vi "IMAQ ROI Type to MSC ROI Type.vi"(0 "IMAQ ROI Type":u32(ring)=4 items=["No Selection", "Point", "Line", "Rectangle", "Oval", "Polygon", "Freehand Region", "Annulus", "Unused2", "Unused3", "Broken Line", "Freehand Line", "Rotated Rectangle"], 11 "error in (no error)":errorcluster) -> (4 "MSC ROI Type":T1 items=["Point", "Line", "Rectangle", "Oval", "Freehand / Polygon"], 15 "error out":errorcluster)   [LabVIEW 2014]
doc: "Conversion from MSC Picture type to IMAQ type"
uses:
  MSC Image_class/controls/ROI Type.ctl
  MSC Image_class/MSC Image.lvclass
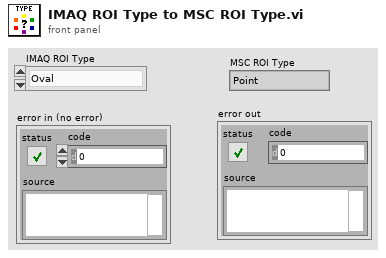
[diagram p1: front panel]
types:
  T1 = typedef "MSC Image.lvclass/ROI Type.ctl" = u16
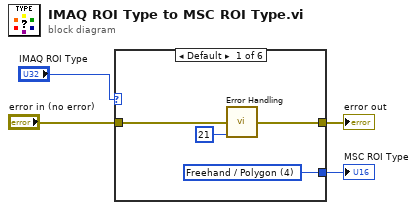
[diagram p0: block diagram]
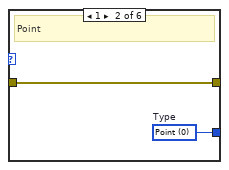
[diagram p2: hidden frame]
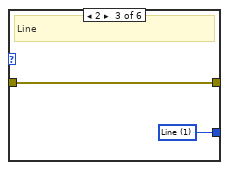
[diagram p3: hidden frame]
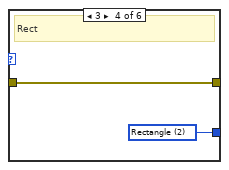
[diagram p4: hidden frame]
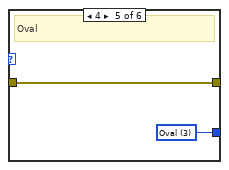
[diagram p5: hidden frame]
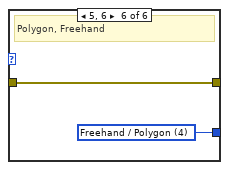
[diagram p6: hidden frame]
diagram:
  n1 = case shown="Default" "IMAQ ROI Type" {
    tunnel: "error in (no error)" -> [w5 w10 w12 w14 w15 w18]
    tunnel: [w6 w10 w12 w14 w15 w18] -> w2
    tunnel: [w8 w9 w11 w13 w16 w17] -> w3
    frame Default {
      w8 = T1 4 items=["Point", "Line", "Rectangle", "Oval", "Freehand / Polygon"] ("Type")
      n2 = call "Error Handling.vi"("error in (no error)"=w5, "return type"=21 ("code")) -> ("error out"=w6:errorcluster)  [unwired: 12 in, 1 out]
    }
    frame 1 {
      w9 = T1 0 items=["Point", "Line", "Rectangle", "Oval", "Freehand / Polygon"]  # Type
      # "Point"
    }
    frame 2 {
      w11 = T1 1 items=["Point", "Line", "Rectangle", "Oval", "Freehand / Polygon"] ("Type")
      # "Line"
    }
    frame 3 {
      w13 = T1 2 items=["Point", "Line", "Rectangle", "Oval", "Freehand / Polygon"] ("Type")
      # "Rect"
    }
    frame 4 {
      w16 = T1 3 items=["Point", "Line", "Rectangle", "Oval", "Freehand / Polygon"] ("Type")
      # "Oval"
    }
    frame 5, 6 {
      w17 = T1 4 items=["Point", "Line", "Rectangle", "Oval", "Freehand / Polygon"] ("Type")
      # "Polygon, Freehand"
    }
  }
  "error out" <- w2
  "MSC ROI Type" <- w3
